vi "İbrahimBerkGelmez.vi"() -> ()   [LabVIEW 2021]
uses:
  <vilib>/LabVIEW Interface for Arduino/Type Defs/Pin Mode.ctl
  <vilib>/LabVIEW Interface for Arduino/LabVIEW Interface for Arduino.lvlib
panel:
  in  "DURDUR":bool
  out "VOLTAJ 1":dbl(knob) scale=0.0..100.0
  in  "SENSÖR PORT":refnum<visa-resource-name>
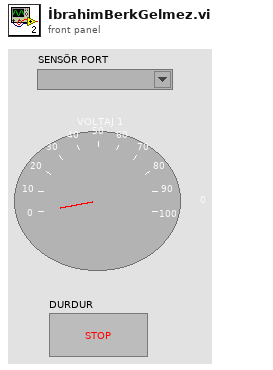
[diagram p1: front panel]
types:
  T1 = typedef "LabVIEW Interface for Arduino.lvlib/Arduino Resource.ctl" = cluster{"VISA resource":refnum<visa-resource-name>, "Board Type":T2, "Connection Type":enum8{"USB / Serial"}, "Bytes Per Packet (15)":u8}
  T2 = typedef "LabVIEW Interface for Arduino.lvlib/Board Type.ctl" = enum16{"Uno", "Dimuelanove w/Atmega 328", "Mega 2560"}
  T3 = typedef "LabVIEW Interface for Arduino.lvlib/Pin Mode.ctl" = enum8{"Input", "Output"}
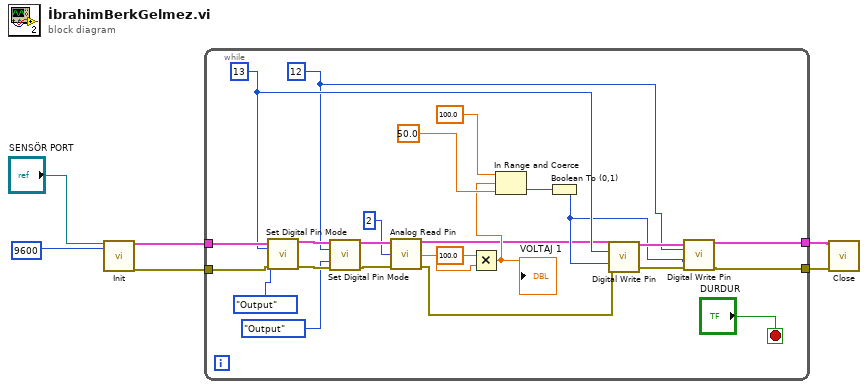
[diagram p0: block diagram]
diagram:
  n1 = call <vilib>:"Init.vi"("VISA resource"="SENSÖR PORT", "Baud Rate (115200)"=u32 9600) -> ("Arduino Resource"=w5:T1, "error out"=w2:errorcluster)  [unwired: 16 in]
  n2 = while {
    tunnel: w5 -> [w31]
    tunnel: [w19] -> w4
    tunnel: [w18] -> w3
    tunnel: w2 -> [w11]
    stop <- "DURDUR" stop-if-true
    w15 = u8 12 ("Digital I/O Pin")
    w16 = u8 13 ("Digital I/O Pin")
    n3 = call <vilib>:"Set Digital Pin Mode.vi"("Arduino Resource"=w31, "Digital I/O Pin"=w16, "Pin Mode (Input)"=Pin_Mode."Output", "error in"=w11) -> ("Arduino Resource"=w30:T1, "error out"=w29:errorcluster)  [unwired: 10 in]
    n4 = call <vilib>:"Set Digital Pin Mode.vi"("Arduino Resource"=w30, "Digital I/O Pin"=w15, "Pin Mode (Input)"=Pin_Mode."Output", "error in"=w29) -> ("Arduino Resource"=w27:T1, "error out"=w26:errorcluster)  [unwired: 10 in]
    n5 = call <vilib>:"Analog Read Pin.vi"("Arduino Resource"=w27, "Analog Input Pin (0)"=u8 2 ("Digital I/O Pin (0)"), "error in"=w26) -> ("Arduino Resource"=w8:T1, "Voltage"=w9:dbl, "error out"=w7:errorcluster)  [unwired: 10 in]
    n6 = Multiply(x=100.0 ("y"), y=w9) -> (x*y=w22:dbl)
    "VOLTAJ 1" <- w22
    n7 = In Range and Coerce(upper limit=100.0, x=w22, lower limit=50.0) -> (In Range?=w13:bool)  [unwired: 1 out]
    n8 = Boolean To (0,1)(Boolean=w13) -> (0, 1=w14:i16)
    n9 = call <vilib>:"Digital Write Pin.vi"("Arduino Resource"=w8, "Digital I/O Pin (0)"=w16, "Value (0)"=w14, "error in"=w7) -> ("Arduino Resource"=w21:T1, "error out"=w20:errorcluster)  [unwired: 10 in]
    n10 = call <vilib>:"Digital Write Pin.vi"("Arduino Resource"=w21, "Digital I/O Pin (0)"=w15, "Value (0)"=w14, "error in"=w20) -> ("Arduino Resource"=w19:T1, "error out"=w18:errorcluster)  [unwired: 10 in]
  }
  n11 = call <vilib>:"Close.vi"("Arduino Resource"=w4, "error in"=w3) -> ()  [unwired: 13 in, 1 out]
